vi "IMAQdx Get Driver Version.vi"(8 "error in":errorcluster) -> (0 "error out":errorcluster, 3 "Driver Version":u32=16777216 format="%08x")   [LabVIEW 2020, in "NI_Vision_Acquisition_Software.lvlib"]
doc: "Returns the current version of the driver."
uses:
  NI_Vision_Acquisition_Software.lvlib
  niimaqdx.dll
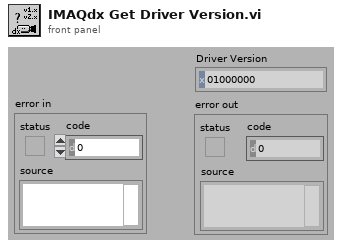
[diagram p1: front panel]
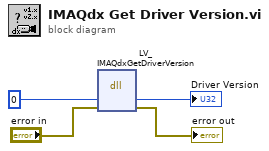
[diagram p0: block diagram]
diagram:
  n1 = dll-call lib="niimaqdx.dll" fn="LV_IMAQdxGetDriverVersion"("driverVersion"=u32 0, "error in"="error in") -> ("driverVersion"=→"Driver Version":u32, "error in"=→"error out":errorcluster)  [unwired: 4 in, 2 out]
